vi "Max Search.vi"() -> ()   [LabVIEW 2025]
panel:
  out "Random Number":dbl
  out "Max":dbl
  in  "Number of Iterations":i32 min=0 step=1
  out "Iteration Count":i32
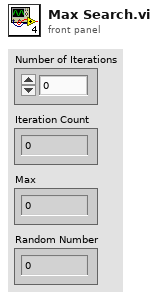
[diagram p1: front panel]
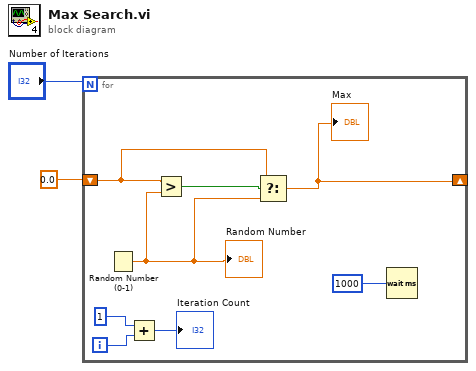
[diagram p0: block diagram]
diagram:
  n1 = for {
    N: "Number of Iterations" -> [_]
    shift-right: [w3] -> _
    shift-left: 0.0 -> [w4]
    i -> [w9]
    n2 = Random Number (0-1)() -> (number: 0 to 1=w5:dbl)
    "Random Number" <- w5
    n3 = Add(x=1, y=w9) -> (x+y=→"Iteration Count":i32)
    n4 = Greater?(x=w4, y=w5) -> (0:w6:bool)
    n5 = Select(t=w4, s=w6, f=w5) -> (s? t:f=w3:dbl)
    "Max" <- w3
    n6 = Wait (ms)(milliseconds to wait=u32 1000) -> ()  [unwired: 1 out]
  }
